vi "Begin.vi"(11 "Image Size":T1=enum."160x120") -> (0 "error out":errorcluster)   [LabVIEW 2012]
doc: "Called before other user functions, this VI is expected to open initial I/O refnums, load in file data, and do all program initialization. Notice that the <B>error out</B> terminal is simply used for data flow. Wiring it to other structures or subVIs ensures that this VI runs first."
uses:
  <vilib>/Rock Robotics/WPI/Camera/WPI_CameraWhite Balance Values.ctl
  <vilib>/Rock Robotics/WPI/Camera/WPI_CameraExposure Values.ctl
  <vilib>/Rock Robotics/WPI/Camera/WPI_CameraFrameRate.ctl
  Robot Global Data.vi
  <vilib>/Rock Robotics/WPI/DriverStation/WPI_DriverStationRobotMode2.ctl
  <vilib>/Rock Robotics/WPI/Camera/WPI_CameraImageSize.ctl
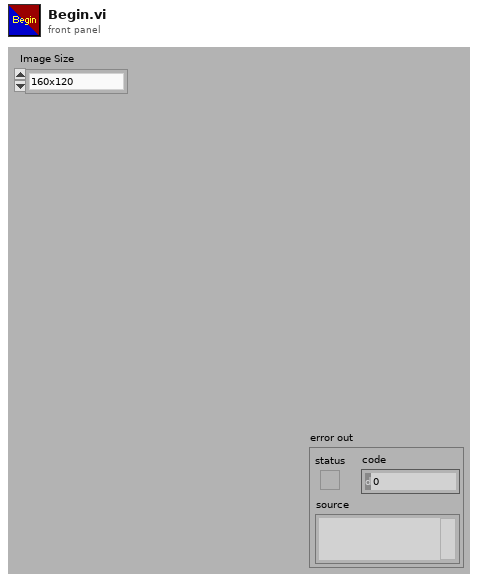
[diagram p1: front panel]
types:
  T1 = typedef "WPI_CameraImageSize.ctl" = enum16{"640x480", "320x240", "160x120"}
  T2 = typedef "WPI_DriverStationRobotMode2.ctl" = enum16{"Autonomous Disabled", "Autonomous Enabled", "Teleop Disabled", "Teleop Enabled", "Timeout", "Finish", "Test Disabled", "Test Enabled"}
  T3 = typedef "WPI_CameraFrameRate.ctl" = u32
  T4 = typedef "WPI_CameraExposure Values.ctl" = enum16{"Auto", "Flicker-free 50 Hz", "Flicker-free 60 Hz", "Hold current"}
  T5 = typedef "WPI_CameraWhite Balance Values.ctl" = enum16{"Auto", "Fixed indoor", "Fixed outdoor 1", "Fixed outdoor 2", "Fixed fluorescent 1", "Fixed fluorescent 2", "Hold current"}
  T6 = typedef "WPI_CameraDevRef.ctl" = cluster{"Camera Address":string, "CameraStatus":errorcluster, "Acquire Image Notifier":refnum<notifier>}
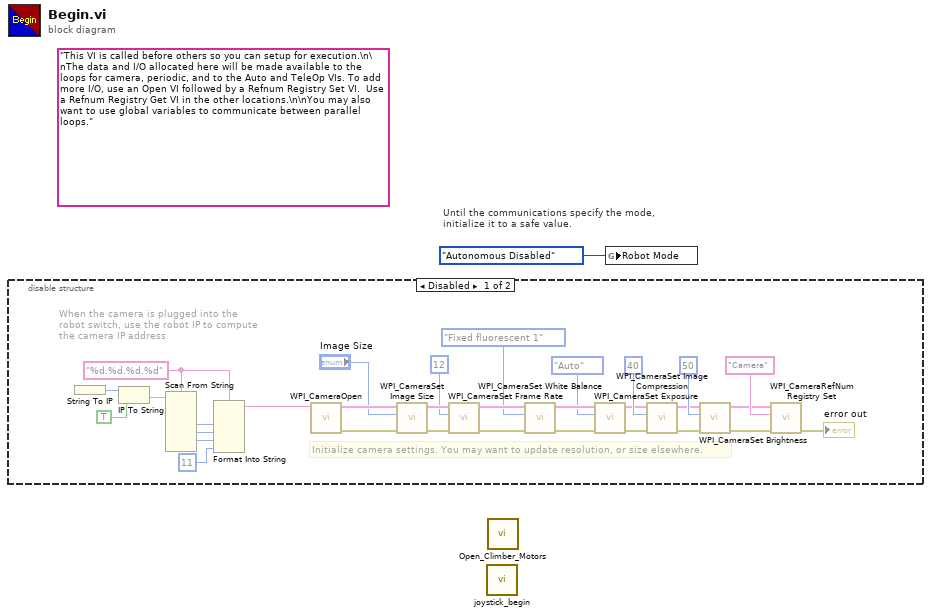
[diagram p0: block diagram]
diagram:
  (unwired) "This VI is called before others so you can setup for execution.\n\nThe data and I/O allocated here will be made available to the loops for camera, periodic, and to the Auto and TeleOp VIs. To add more I/O, use an Open VI followed by a Refnum Registry Set VI.  Use a Refnum Registry Get VI in the other locations.\n\nYou may also want to use global variables to communicate between parallel loops."
  # "Until the communications specify the mode,\ninitialize it to a safe value."
  n1 = disable-structure shown="Disabled" {
    frame Disabled {
      w4 = "%d.%d.%d.%d" ("format string")
      # "When the camera is plugged into the\nrobot switch, use the robot IP to compute\nthe camera IP address"
      # "Initialize camera settings. You may want to update resolution, or size elsewhere."
      n2 = String To IP() -> (0:w11:u32)  [unwired: 1 in]
      n3 = IP To String(1:TRUE ("dot notation? (F)"), 2:w11) -> (0:w9:string)
      n4 = Scan From String(format string=w4, input string=w9) -> (output 1=w8:i32, output 2=w7:i32, output 3=w6:i32)  [unwired: 7 in, 3 out]
      n5 = Format Into String(format string=w4, w8, w7, w6, 11 ("Compression")) -> (resulting string=w3:string)  [unwired: 2 in, 1 out]
      n6 = call <vilib>:"WPI_CameraOpen.vi"("Camera Address"=w3) -> ("error out"=w23:errorcluster, "CameraDevRef"=w24:T6)  [unwired: 1 in, 8 out]
      n7 = call <vilib>:"WPI_CameraSet Image Size.vi"("error in (no error)"=w23, "Image Size"="Image Size", "CameraDevRef"=w24) -> ("error out"=w22:errorcluster, "CameraDevRef Out"=w25:T6)  [unwired: 7 out]
      n8 = call <vilib>:"WPI_CameraSet Frame Rate.vi"("error in (no error)"=w22, "Frame Rate (fps)"=T3 12, "CameraDevRef"=w25) -> ("error out"=w21:errorcluster, "CameraDevRef Out"=w27:T6)  [unwired: 7 out]
      n9 = call <vilib>:"WPI_CameraSet White Balance.vi"("error in (no error)"=w21, "White Balance"=WPI_CameraWhite_Balance_Values."Fixed fluorescent 1", "CameraDevRef"=w27) -> ("error out"=w20:errorcluster, "CameraDevRef Out"=w26:T6)  [unwired: 7 out]
      n10 = call <vilib>:"WPI_CameraSet Exposure.vi"("error in (no error)"=w20, "Exposure"=WPI_CameraExposure_Values."Auto", "CameraDevRef"=w26) -> ("error out"=w19:errorcluster, "CameraDevRef Out"=w29:T6)  [unwired: 7 out]
      n11 = call <vilib>:"WPI_CameraSet Image Compression.vi"("error in (no error)"=w19, "Compression"=40, "CameraDevRef"=w29) -> ("error out"=w18:errorcluster, "CameraDevRef Out"=w28:T6)  [unwired: 7 out]
      n12 = call <vilib>:"WPI_CameraSet Brightness.vi"("error in (no error)"=w18, "Brightness"=50, "CameraDevRef"=w28) -> ("error out"=w16:errorcluster, "CameraDevRef Out"=w17:T6)  [unwired: 7 out]
      n13 = call <vilib>:"WPI_CameraRefNum Registry Set.vi"("error in (no error)"=w16, "refnum name"="Camera", "CameraDevRef"=w17) -> ("error out"=→"error out":errorcluster)  [unwired: 8 out]
    }
    frame Enabled {
    }
  }
  n14 = call "joystick_begin.vi"() -> ()  [unwired: 11 in, 1 out]
  n15 = call "Open_Climber_Motors.vi"() -> ()  [unwired: 10 in]
  n16 = global write "Robot Global Data.vi" "Robot Mode"(WPI_DriverStationRobotMode2."Autonomous Disabled" ("Robot Mode")) -> ()
